vi "waitStatusSweepingStarted.vi"(8 "error in (no error)":errorcluster, 11 "Instrument.Lockin in":refnum<class "Instrument.Lockin.lvclass">) -> (0 "error out":errorcluster, 3 "Instrument.Lockin out":refnum<class "Instrument.Lockin.lvclass">)   [LabVIEW 2019, in "Instrument.Lockin.lvclass"]
uses:
  Instrument.Lockin.lvclass
  Lockin.DAQ/Typedefs/State-enum.ctl
  Lockin.DAQ/Lockin.DAQ.lvclass
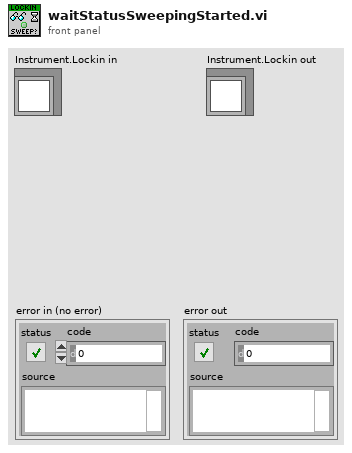
[diagram p1: front panel]
types:
  T1 = typedef "Lockin.DAQ.lvclass/State-enum.ctl" = enum16{"idle", "created", "started", "stopped", "sweeping"}
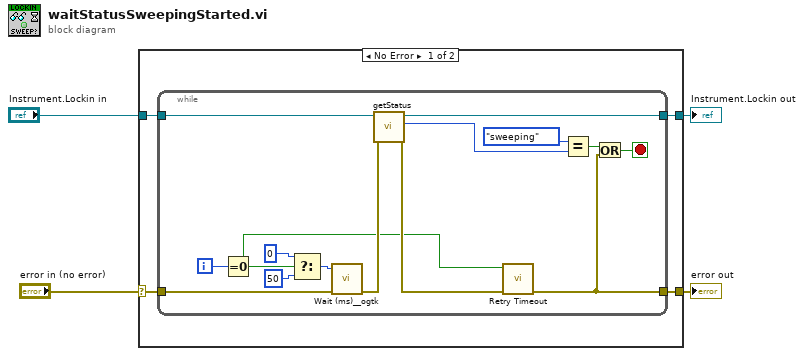
[diagram p0: block diagram]
diagram:
  n1 = case shown="No Error" "error in (no error)" {
    selector: "error in (no error)" -> [w5 w24]
    tunnel: [w8 w24] -> w4
    tunnel: [w7 w25] -> w3
    tunnel: "Instrument.Lockin in" -> [w6 w25]
    frame No Error {
      n2 = while {
        tunnel: w5 -> [w23]
        tunnel: [w12] -> w8
        tunnel: w6 -> [w18]
        tunnel: [w17] -> w7
        i -> [w10]
        stop <- w22 stop-if-true
        n3 = Equal To 0?(x=w10) -> (x = 0?=w9:bool)
        n4 = Select(t=u32 0, s=w9, f=u32 50 ("milliseconds to wait")) -> (s? t:f=w19:u32)
        n5 = call <userlib>:"Wait (ms)__ogtk.vi"("error in (no error)"=w23, "milliseconds to wait"=w19) -> ("error out"=w13:errorcluster)  [unwired: 8 in, 1 out]
        n6 = call "getStatus.vi"("error in (no error)"=w13, "Instrument.Lockin"=w18) -> ("error out"=w11:errorcluster, "Status"=w15:T1, "Instrument.Lockin"=w17:refnum<class "Instrument.Lockin.lvclass">)  [unwired: 7 in]
        n7 = call "Retry Timeout.vi"("error in (no error)"=w11, "reset"=w9) -> ("error out"=w12:errorcluster)  [unwired: 8 in, 1 out]
        n8 = Equal?(x=State-enum."sweeping" ("Status"), y=w15) -> (x = y?=w14:bool)
        n9 = Or(x=w14, y=w12) -> (x .or. y?=w22:bool)
      }
    }
    frame Error {
    }
  }
  "error out" <- w4
  "Instrument.Lockin out" <- w3
